vi "AquisicaoGeral.vi"() -> ()   [LabVIEW 2011]
panel:
  out "Waveform Chart":dynamicdata(graph)
  in  "stop":bool
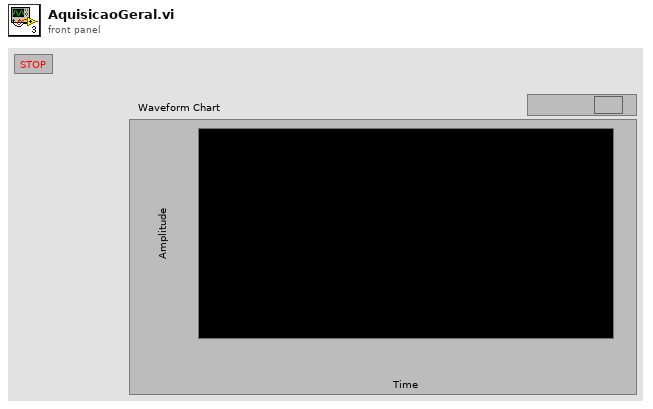
[diagram p1: front panel]
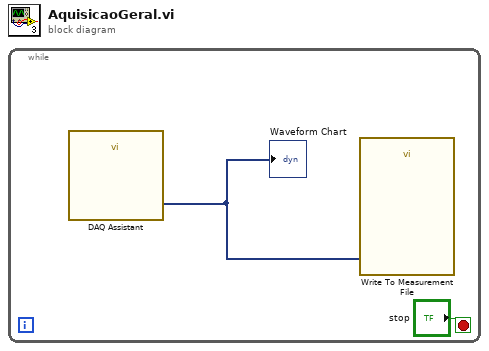
[diagram p0: block diagram]
diagram:
  n1 = while {
    stop <- "stop" stop-if-true
    n2 = call "DAQ Assistant"() -> ("data"=w1:dynamicdata)  [unwired: 16 in, 3 out]
    "Waveform Chart" <- w1
    n3 = call "Write To Measurement File"("Signals"=w1) -> ()  [unwired: 16 in, 3 out]
  }
